vi "Insert Created.vi"(7 "Metric Name":string, 8 "error in (no error)":errorcluster, 11 "Counter in":refnum<class "Counter.lvclass">) -> (0 "error out":errorcluster, 3 "Counter out":refnum<class "Counter.lvclass">)   [LabVIEW 2020, in "Metrics.lvlib" / "Counter.lvclass"]
uses:
  Counter.lvclass
  gauge/Gauge.lvclass
  C:/Github-locals/PromVIEW/src/metrics/metric/Metric.lvclass
  metric/Metric.lvclass/Metric.ctl
  Counter.lvclass/Counter.ctl
  metric/Write Name.vi
  metric/Validate Name.vi
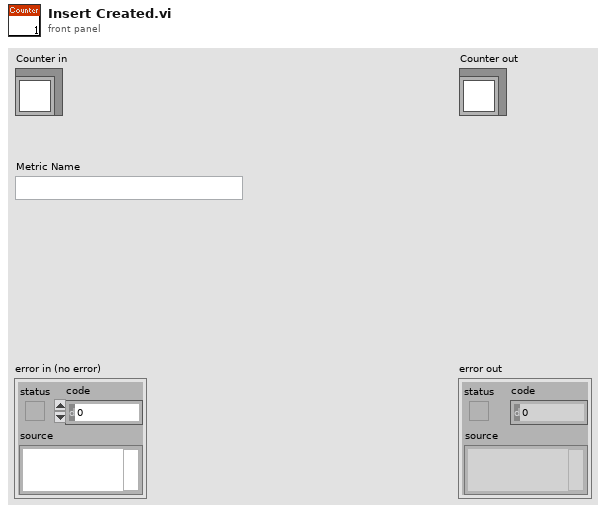
[diagram p1: front panel]
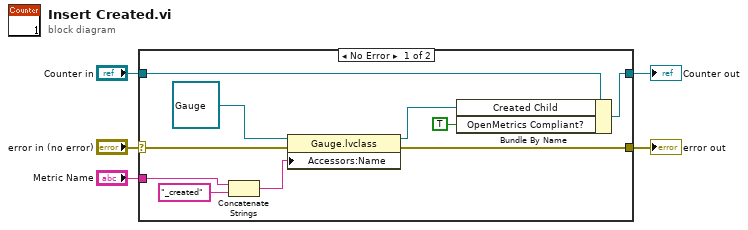
[diagram p0: block diagram]
diagram:
  n1 = case shown="No Error" "error in (no error)" {
    selector: "error in (no error)" -> [w8 w17]
    tunnel: [w7 w17] -> w4
    tunnel: [w14 w16] -> w2
    tunnel: "Counter in" -> [w15 w16]
    tunnel: "Metric Name" -> [w11 _]
    frame No Error {
      n2 = Concatenate Strings(w11, "_created" ("string")) -> (w10:string)
      n3 = property class="Gauge.lvclass"(reference=refnum<class "Gauge.lvclass"> refnum ("Metrics.lvlib:Gauge.lvclass"), error in=w8, "Accessors:Name"=w10) -> (reference out=w9:refnum<class "Gauge.lvclass">, error out=w7:errorcluster)
      n4 = Bundle By Name(cluster=w15, "Created Child"=w9, "OpenMetrics Compliant?"=TRUE) -> (w14:refnum<class "Counter.lvclass">)
    }
    frame Error {
    }
  }
  "error out" <- w4
  "Counter out" <- w2
